vi "Create a New Document.vi"(7 "Document Type":refnum<class "npoiDocument.lvclass">, 8 "error in (no error)":errorcluster, 11 "Document Path":path) -> (0 "error out":errorcluster, 3 "Document out":refnum<class "npoiDocument.lvclass">)   [LabVIEW 2017, in "NPOI_Document.lvlib" / "npoiDocument.lvclass"]
doc: "Creates a new <b>Document out</b>,of the <b>Document Type</b> file format, at the <b>Document Path</b> location if its provided. Use save to persist your changes.\n\nNotes:\n - If the <b>Document Path</b> already contains a docuement with the same name then that file is overwritten without warning."
uses:
  npoiDocument.lvclass
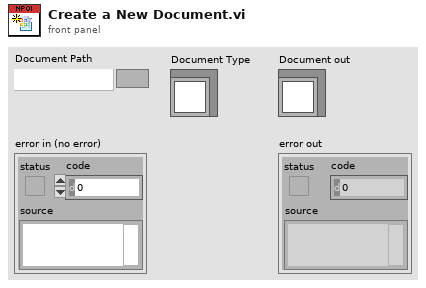
[diagram p1: front panel]
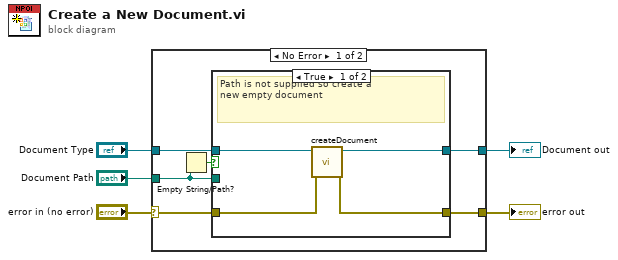
[diagram p0: block diagram]
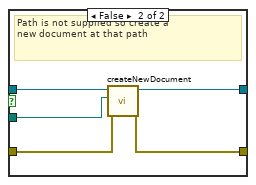
[diagram p2: hidden frame]
diagram:
  n1 = case shown="No Error" "error in (no error)" {
    selector: "error in (no error)" -> [w9 w22]
    tunnel: [w8 w22] -> w4
    tunnel: [w10 w21] -> w2
    tunnel: "Document Type" -> [w11 w21]
    tunnel: "Document Path" -> [w7 _]
    frame No Error {
      n2 = Empty String/Path?(string/path=w7) -> (empty?=w6:bool)
      n3 = case shown="True" w6 {
        tunnel: w11 -> [w15 w20]
        tunnel: [w12 w17] -> w10
        tunnel: w9 -> [w14 w19]
        tunnel: [w13 w18] -> w8
        tunnel: w7 -> [_ w16]
        frame True {
          # "Path is not supplied so create a \nnew empty document"
          n4 = call-dynamic "createDocument.vi"("error in (no error)"=w14, "npoiDocument in"=w15) -> ("error out"=w13:errorcluster, "npoiDocument out"=w12:refnum<class "npoiDocument.lvclass">)  [unwired: 8 in]
        }
        frame False {
          # "Path is not supplied so create a \nnew document at that path"
          n5 = call-dynamic "createNewDocument.vi"("error in (no error)"=w19, "Document Path"=w16, "npoiDocument in"=w20) -> ("error out"=w18:errorcluster, "npoiDocument out"=w17:refnum<class "npoiDocument.lvclass">)  [unwired: 7 in]
        }
      }
    }
    frame Error {
    }
  }
  "error out" <- w4
  "Document out" <- w2
